vi "DatabaseAPI-Connect-SecondaryDb.vi"(8 "error in (no error)":errorcluster, 9 "Database (mdb)  File Path":path=path "C:/Program Files (x86)/ITS/Specification Manager/data/ITSSpecificationDB.udl", 11 "Database-API in":refnum<class "Database-API.lvclass">) -> (0 "error out":errorcluster, 3 "Database-API out":refnum<class "Database-API.lvclass">)   [LabVIEW 2014, in "Database-API.lvclass"]
uses:
  Database-API.lvclass
  Database-API.lvclass/Database-API.ctl
  <vilib>/addons/database/Connection.llb/DB Tools Open Connec (Path).vi
  <vilib>/addons/database/NI_Database_API.lvlib
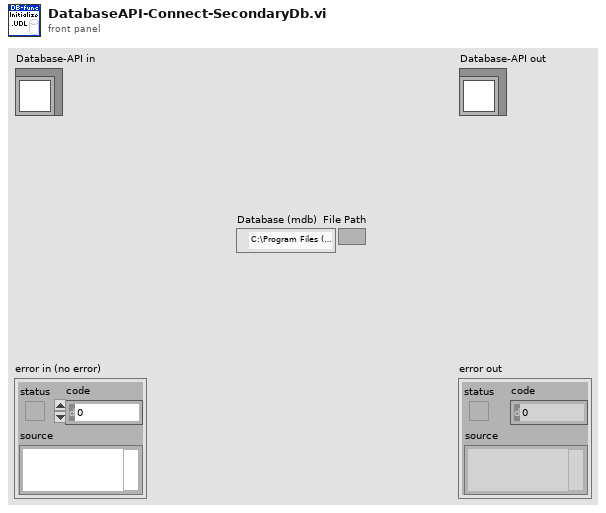
[diagram p1: front panel]
types:
  T1 = typedef "NI_Database_API.lvlib/Conn ObjectReference.ctl" = refnum<k1>
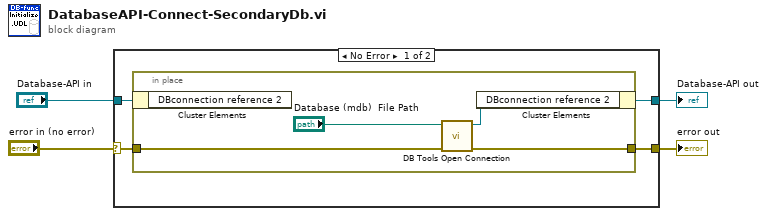
[diagram p0: block diagram]
diagram:
  n1 = case shown="No Error" "error in (no error)" {
    selector: "error in (no error)" -> [w7 w14]
    tunnel: [w6 w14] -> w3
    tunnel: [w5 w13] -> w1
    tunnel: "Database-API in" -> [w8 w13]
    frame No Error {
      n2 = in-place {
        in-place-border: w7 -> [w10]
        in-place-border: [w9] -> w6
        n3 = in-place-cluster #1(w8) -> ()  [unwired: 1 out]
        n4 = call-poly <vilib>:"DB Tools Open Connection.vi"("error in (no error)"=w10, "connection information"="Database (mdb)  File Path") -> ("error out"=w9:errorcluster, "connection reference"=w11:T1)  [unwired: 6 in]
        n5 = in-place-cluster #1("DBconnection reference 2"=w11) -> (w5:refnum<class "Database-API.lvclass">)
      }
    }
    frame Error {
    }
  }
  "error out" <- w3
  "Database-API out" <- w1
